vi "总磷测量流程.vi"(11 "控制命令":T1(ring)) -> ()   [LabVIEW 2016, in "斯坦道总磷.lvlib"]
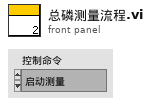
[diagram p1: front panel]
types:
  T1 = enum16{"启动测量", "标样核查", "零点核查", "跨度核查", "空白测试", "平行样测试", "加标回收", "空白校准", "标样校准", "初始化（清洗）", "停止测试", "仪器重启", "校时", "模式设置", "测量间隔设置"}
  T2 = cluster{"时间标识":timestamp, "设备":string, "日志信息":string, "流程参数":string}
  T3 = cluster{"站号":u16, "量程切换":enum32{"H", "L", "AUTO"}, "控制命令":enum16{"启动测量", "标样核查", "零点核查", "跨度核查", "空白测试", "平行样测试", "加标回收", "空白校准", "标样校准", "初始化（清洗）", "停止测试", "仪器重启", "校时", "模式设置", "测量间隔设置"}, "模式设置":enum16{"待机", "连续模式", "周期模式", "定点模式", "受控模式", "手动模式"}, "测量间隔":u16}
  T4 = cluster{"系统时间":timestamp, "工作状态":enum16{"空闲", "水样测试", "标样核查", "零点核查", "跨度核查", "空白测试", "平行样测试", "加标回收", "空白校准", "标样校准", "初始化（清洗）"}, "测量模式":enum16{"待机", "连续模式", "周期模式", "定点模式", "受控模式", "手动模式"}, "告警代码":u16, "故障代码":u16, "日志代码":u16, "软件版本":u16, "F0":sgl, "F1":sgl, "F2":sgl, "F3":sgl, "T":sgl, "H":sgl, "id":u16, "flowid":u16, "量程":u16, "总磷控温温度1":sgl, "营养盐控温温度2":sgl, "ADC":sgl}
  T5 = cluster{"水样测试量程模式":enum16{"H", "L", "AUTO"}, "空白核查量程模式":enum16{"H", "L", "AUTO"}, "跨度核查量程模式":enum16{"H", "L", "AUTO"}}
  T6 = enum16{"空闲", "水样测试", "标样核查", "零点核查", "跨度核查", "空白测试", "平行样测试", "加标回收", "空白校准", "标样校准", "初始化（清洗）"}
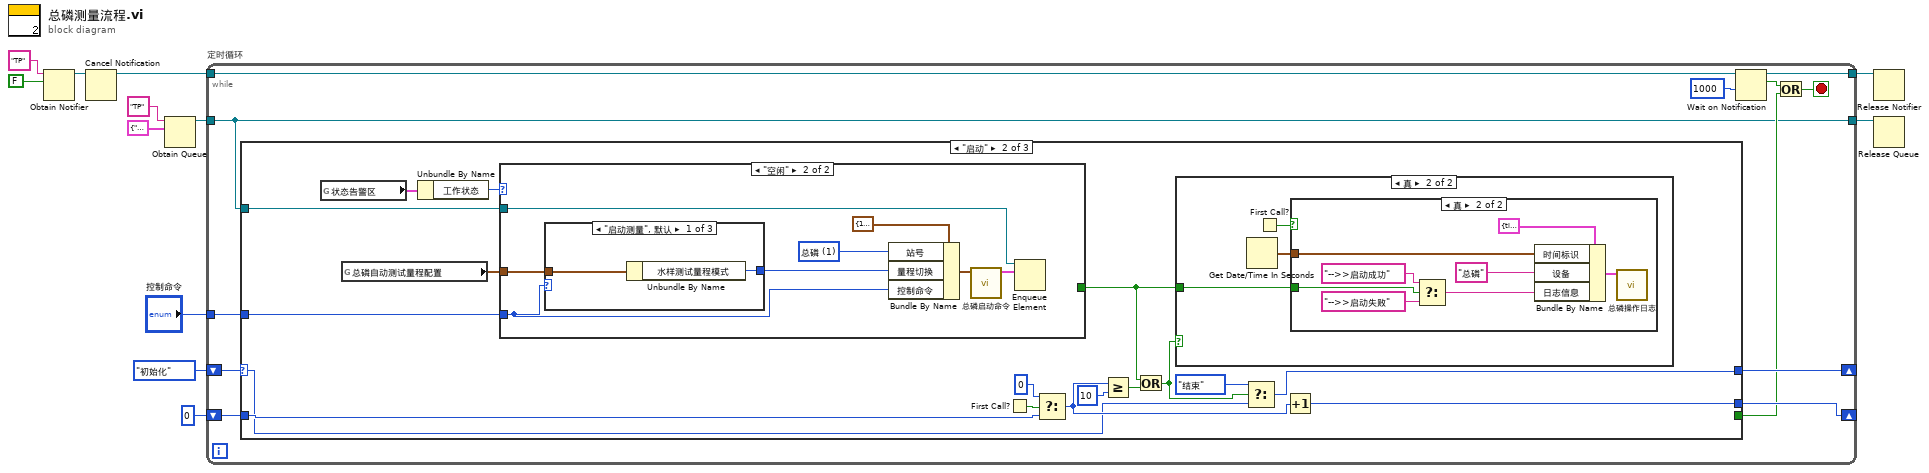
[diagram p0: block diagram]
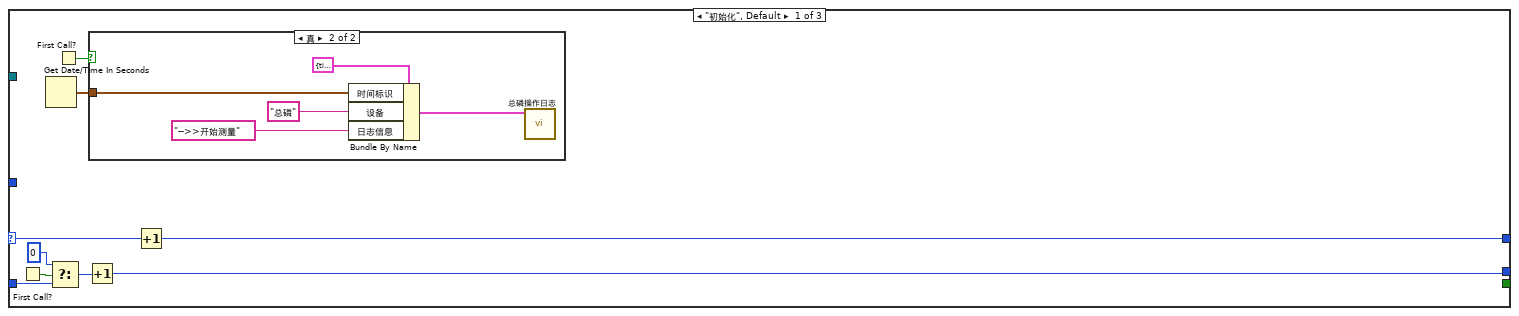
[diagram p2: hidden frame]
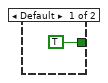
[diagram p6: hidden frame]
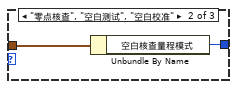
[diagram p7: hidden frame]
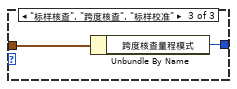
[diagram p8: hidden frame]
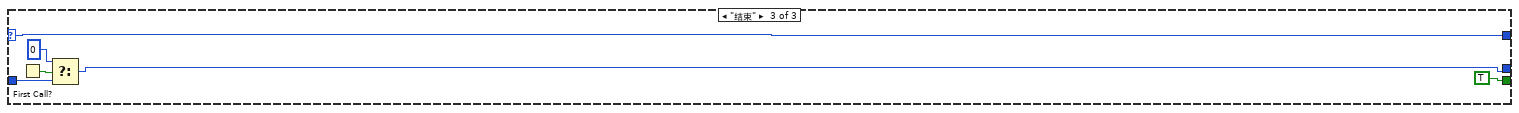
[diagram p9: hidden frame]
diagram:
  n1 = Obtain Notifier(name (unnamed)="TP" ("名称（未命名）"), notification data type=FALSE) -> (notifier out=w7:refnum<notifier>)  [unwired: 2 in, 2 out]
  n2 = Cancel Notification(0:w7) -> (8:w6:refnum<notifier>)  [unwired: 1 in, 2 out]
  n3 = Obtain Queue(name (unnamed)="TP" ("名称（未命名）"), element data type=cluster{"命令":string, "data":variant} {"命令"="", "data"=variant}) -> (queue out=w10:refnum<queue>)  [unwired: 3 in, 2 out]
  n4 = while "定时循环" {
    tunnel: w10 -> [w13]
    tunnel: w6 -> [w24]
    tunnel: "控制命令" -> [w19]
    shift-right: [w18] -> _
    shift-left: enum16{"初始化", "启动", "结束"}."初始化" -> [w20]
    shift-right: [w16] -> _
    shift-left: 0 -> [w17]
    tunnel: [w14] -> w2
    tunnel: [w13] -> w3
    stop <- w21 stop-if-true
    n5 = case shown="\"启动\"" w20 {
      selector: w20 -> [w31 w44 w87]
      tunnel: w19 -> [_ w55 _]
      tunnel: w13 -> [_ w54 _]
      tunnel: [w30 w45 w87] -> w18
      tunnel: w17 -> [w28 w49 w84]
      tunnel: [w25 w48 w83] -> w16
      tunnel: [_ _ TRUE] -> w15
      frame "初始化", Default {
        n6 = First Call?() -> (First Call?: T/F=w29:bool)
        n7 = Get Date/Time In Seconds() -> (seconds since 1Jan1904=w33:timestamp)
        n8 = Select(t=0, s=w29, f=w28) -> (s? t:f=w26:i32)
        n9 = First Call?() -> (First Call?: T/F=w32:bool)
        n10 = Increment(x=w26) -> (x+1=w25:i32)
        n11 = case shown="真" w32 {
          tunnel: w33 -> [_ w37]
          frame False {
          }
          frame True {
            n12 = Bundle By Name(cluster=T2 {"时间标识"=timestamp(0 s since 1904-01-01), "设备"="", "日志信息"="", "流程参数"=""} ("data in"), "时间标识"=w37, "设备"="总磷", "日志信息"="-->>开始测量") -> (w38:T2)
            n13 = call "总磷操作日志.vi"("data in"=w38) -> ()  [unwired: 11 in]
          }
        }
        n14 = Increment(x=w31) -> (x+1=w30:enum16{"初始化", "启动", "结束"})
      }
      frame "启动" {
        n15 = global read "VAR总磷全局变量.vi" "状态告警区"() -> (w53:T4)
        n16 = global read "总磷断电保存全局变量.vi" "总磷自动测试量程配置"() -> (w39:T5)
        n17 = Unbundle By Name(w53) -> ("工作状态"=w52:T6)
        n18 = case shown="\"空闲\"" w52 {
          tunnel: w39 -> [_ w73]
          tunnel: w55 -> [_ w68]
          tunnel: w54 -> [_ w72]
          tunnel: [TRUE _] -> w40
          frame Default {
          }
          frame "空闲" {
            w71 = u16 1 items=["总磷"=1, "总氮"=2, "氨氮"=3] ("站号")
            n19 = case shown="\"启动测量\", 默认" w68 {
              tunnel: w73 -> [w77 w79 w81]
              tunnel: [w76 w78 w80] -> w75
              frame "启动测量", Default {
                n20 = Unbundle By Name(w77) -> ("水样测试量程模式"=w76:enum16{"H", "L", "AUTO"})
              }
              frame "零点核查", "空白测试", "空白校准" {
                n21 = Unbundle By Name(w79) -> ("空白核查量程模式"=w78:enum16{"H", "L", "AUTO"})
              }
              frame "标样核查", "跨度核查", "标样校准" {
                n22 = Unbundle By Name(w81) -> ("跨度核查量程模式"=w80:enum16{"H", "L", "AUTO"})
              }
            }
            n23 = Bundle By Name(cluster=T3 {"站号"=1, "量程切换"=enum."AUTO", "控制命令"=enum."启动测量", "模式设置"=enum."待机", "测量间隔"=0} ("参数"), "站号"=w71, "量程切换"=w75, "控制命令"=w68) -> (w69:T3)
            n24 = call "总磷启动命令.vi"("参数"=w69) -> ("启动命令"=w74:cluster{"命令":string, "data":variant})  [unwired: 10 in]
            n25 = Enqueue Element(queue=w72, element=w74) -> ()  [unwired: 2 in, 3 out]
          }
        }
        n26 = First Call?() -> (First Call?: T/F=w51:bool)
        n27 = Select(t=0, s=w51, f=w49) -> (s? t:f=w47:i32)
        n28 = Greater Or Equal?(x=w47, y=10) -> (x >= y?=w43:bool)
        n29 = Or(x=w40, y=w43) -> (x .or. y?=w41:bool)
        n30 = case shown="真" w41 {
          tunnel: w40 -> [_ w56]
          frame False {
          }
          frame True {
            n31 = Get Date/Time In Seconds() -> (seconds since 1Jan1904=w57:timestamp)
            n32 = First Call?() -> (First Call?: T/F=w58:bool)
            n33 = case shown="真" w58 {
              tunnel: w57 -> [_ w65]
              tunnel: w56 -> [_ w62]
              frame False {
              }
              frame True {
                n34 = Select(t="-->>启动成功" ("日志信息"), s=w62, f="-->>启动失败" ("日志信息")) -> (s? t:f=w59:string)
                n35 = Bundle By Name(cluster=T2 {"时间标识"=timestamp(0 s since 1904-01-01), "设备"="", "日志信息"="", "流程参数"=""} ("data in"), "时间标识"=w65, "设备"="总磷", "日志信息"=w59) -> (w66:T2)
                n36 = call "总磷操作日志.vi"("data in"=w66) -> ()  [unwired: 11 in]
              }
            }
          }
        }
        n37 = Select(t=enum16{"初始化", "启动", "结束"}."结束", s=w41, f=w44) -> (s? t:f=w45:enum16{"初始化", "启动", "结束"})
        n38 = Increment(x=w47) -> (x+1=w48:i32)
      }
      frame "结束" {
        n39 = First Call?() -> (First Call?: T/F=w86:bool)
        n40 = Select(t=0, s=w86, f=w84) -> (s? t:f=w83:i32)
      }
    }
    n41 = Wait on Notification(notifier=w24, timeout in ms (-1)=1000 ("超时毫秒(-1)")) -> (notifier out=w14:refnum<notifier>, notification=w22:bool)  [unwired: 2 in, 2 out]
    n42 = Or(x=w22, y=w15) -> (x .or. y?=w21:bool)
  }
  n43 = Release Notifier(notifier=w2) -> ()  [unwired: 2 in, 3 out]
  n44 = Release Queue(queue=w3) -> ()  [unwired: 2 in, 3 out]
